vi "ucno_function and gradient.vi"(6 "output control":T3, 7 "function and data":T1, 8 "error in (no error)":errorcluster, 11 "X":dbl[](array[numeric])) -> (0 "error out":errorcluster, 1 "number of function calls":i32, 2 "gradient":dbl[](array[numeric]), 3 "f(X)":dbl)   [LabVIEW 2014, in "NI_Gmath.lvlib"]
uses:
  NI_Gmath.lvlib
  ucno_output select.ctl
  ucno_user function ref and data.ctl
  ucno_user objective function ref.ctl
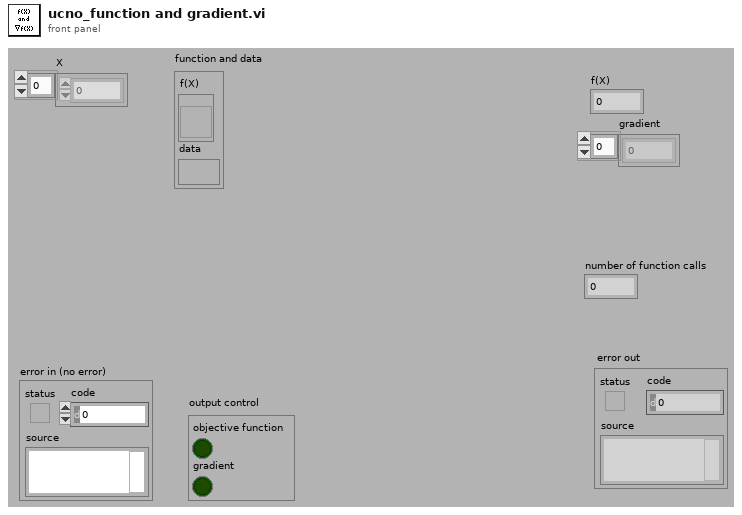
[diagram p1: front panel]
types:
  T1 = typedef "NI_Gmath.lvlib/ucno_user function ref and data.ctl" = cluster{"f(X)":T2, "data":variant}
  T2 = typedef "NI_Gmath.lvlib/ucno_user objective function ref.ctl" = refnum<vi>
  T3 = typedef "NI_Gmath.lvlib/ucno_output select.ctl" = cluster{"objective function":bool, "gradient":bool}
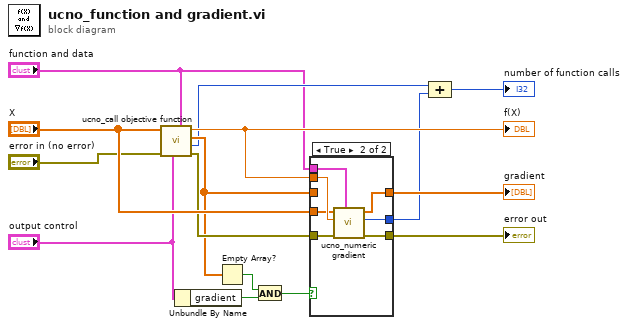
[diagram p0: block diagram]
diagram:
  n1 = call "ucno_call objective function.vi"("function and data"="function and data", "output control"="output control", "error in (no error)"="error in (no error)", "X"="X") -> ("error out"=w9:errorcluster, "number of function evaluations"=w4:i32, "gradient"=w5:dbl[], "f(X)"=w13:dbl)  [unwired: 4 in]
  "f(X)" <- w13
  n2 = Unbundle By Name("output control") -> ("gradient"=w8:bool)
  n3 = Empty Array?(array=w5) -> (empty?=w7:bool)
  n4 = And(x=w7, y=w8) -> (x .and. y?=w6:bool)
  n5 = case shown="True" w6 {
    tunnel: "X" -> [_ w19]
    tunnel: w13 -> [_ w24]
    tunnel: w9 -> [w16 w23]
    tunnel: [w17 w20] -> w12
    tunnel: [w16 w22] -> w11
    tunnel: [_ w21] -> w10
    tunnel: w5 -> [w17 _]
    tunnel: "function and data" -> [_ w18]
    frame False {
    }
    frame True {
      n6 = call "ucno_numeric gradient.vi"("function and data"=w18, "error in (no error)"=w23, "f(X)"=w24, "X"=w19) -> ("error out"=w22:errorcluster, "number of function evaluations"=w21:i32, "gradient"=w20:dbl[])  [unwired: 5 in]
    }
  }
  "gradient" <- w12
  "error out" <- w11
  n7 = Compound Arithmetic op=ADD(w4, w10) -> (→"number of function calls":i32)
